vi "Offset Change.vi"(2 "Offsets":dbl[](array[numeric]) format="%^_3e", 3 "Configured Inst Input":T1[](array[typedef]) {"Private"."Offset" format="%^_3e"; "Private"."Scale Factors" format="%^_3e"}) -> (0 "Configured Inst dup":T1[](array[typedef]) {"Private"."Offset" format="%^_3e"; "Private"."Scale Factors" format="%^_3e"})   [LabVIEW 2019]
uses:
  Sub Controls/Instrument Properties.ctl
  Sub Controls/Public.ctl
  Sub Controls/Private.ctl
  Sub Controls/Instrument Ref.ctl
  Sub Controls/SystemCheckBox-resize.ctl
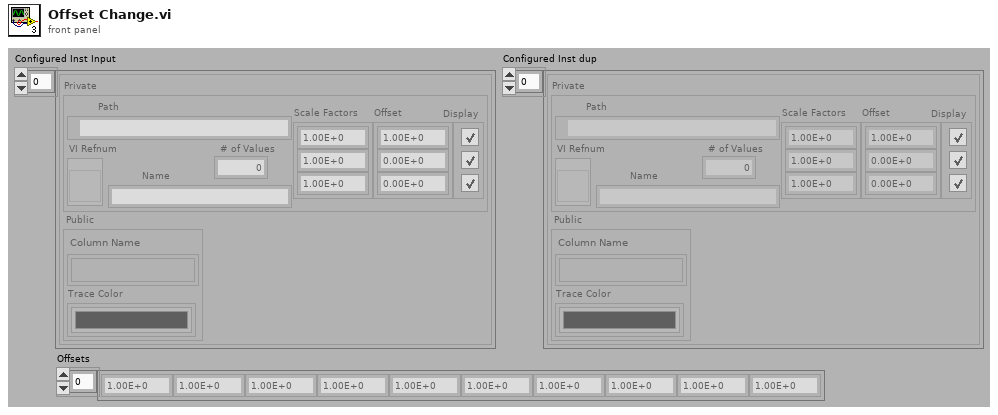
[diagram p1: front panel]
types:
  T1 = typedef "Instrument Properties.ctl" = cluster{"Public":T2, "Private":T3}
  T2 = typedef "Public.ctl" = cluster{"Column Name":string[], "Trace Color":u32[]}
  T3 = typedef "Private.ctl" = cluster{"Path":path, "VI Refnum":T4, "Name":string, "# of Values":i32, "Scale Factors":dbl[], "Display":T5[], "Offset":dbl[]}
  T4 = typedef "Instrument Ref.ctl" = refnum<vi>
  T5 = typedef "SystemCheckBox-resize.ctl" = bool
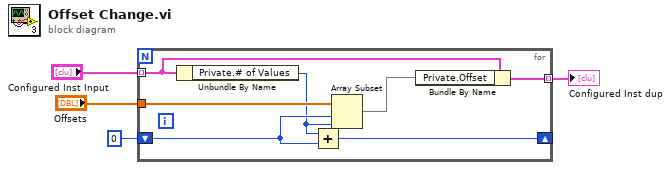
[diagram p0: block diagram]
diagram:
  n1 = for {
    tunnel: "Configured Inst Input" -> [w9] mode=indexing
    shift-right: [w11] -> _
    shift-left: 0 -> [w7]
    tunnel: "Offsets" -> [w10]
    tunnel: [w8] -> w4 mode=indexing
    n2 = Unbundle By Name(w9) -> ("Private.# of Values"=w5:i32)
    n3 = Add(x=w5, y=w7) -> (x+y=w11:i32)
    n4 = Array Subset(array=w10, index=w7, length=w5) -> (w6:dbl[])
    n5 = Bundle By Name(cluster=w9, "Private.Offset"=w6) -> (w8:T1)
  }
  "Configured Inst dup" <- w4
